vi "changeMonitorState.vi"(8 "error in (no error)":errorcluster, 10 "State":u16, 11 "Subnet in":refnum<class "Subnet.lvclass">) -> (0 "error out":errorcluster, 3 "Subnet out":refnum<class "Subnet.lvclass">)   [LabVIEW 2016, in "Subnet.lvclass"]
uses:
  Subnet.lvclass
  Subnet.lvclass/Subnet.ctl
  Common_RT_ILC/ILC/ILC.lvclass/ILC.ctl
  Common_RT_MTILC/MTILC/MTILC.lvclass
  D:/Code/Common_RT_ILC/ILC/ILC.lvclass
  Common_RT_MDILC/MDILC/MDILC.lvclass
  Common_RT_MIILC/MIILC/MIILC.lvclass
  Common_RT_Modbus/IModbus/IModbus.lvclass
  Common_RT_ILC/ILC/ILC.lvclass
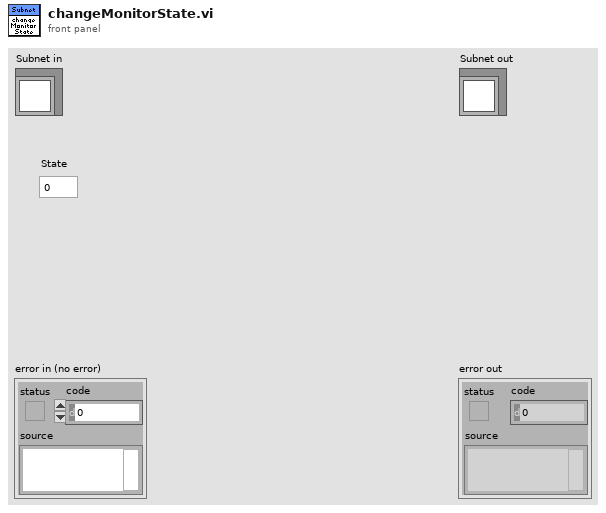
[diagram p1: front panel]
types:
  T1 = typedef "RTILC.lvlib/ILCData.ctl" = cluster{"Constants":T2, "Command":T3, "Telemetry":T5, "Responses":T6, "Timings":T8}
  T2 = typedef "RTILC.lvlib/ILCConstants.ctl" = cluster{"Subnet":u8, "Address":u8}
  T3 = typedef "RTILC.lvlib/ILCCommand.ctl" = cluster{"ILCMode":u16, "TemporaryAddress":u8, "ADCScanRate":T4, "ADCChannel":u8, "ADCOffset":sgl, "ADCSensitivity":sgl}
  T4 = typedef "RTILC.lvlib/ILCScanRates.ctl" = u8
  T5 = typedef "RTILC.lvlib/ILCTelemetry.ctl" = cluster{"UniqueID":u64, "FirmwareType":u8, "NetworkNodeType":u8, "ILCOption":u8, "NetworkNodeOption":u8, "MajorRevision":u8, "MinorRevision":u8, "FirmwareName":string, "ILCMode":u16, "MajorFault":bool, "MinorFault":bool, "FaultOverride":bool, "UniqueIDCRCMismatch":bool, "AppTypeNodeTypeMismatch":bool, "AppMissing":bool, "AppCRCMismatch":bool, "TEDSNotFound":bool, "TEDS1Mismatch":bool, "TEDS2Mismatch":bool, "WatchdogResetDetected":bool, "BrownoutDetected":bool, "EventTrapResetDetected":bool, "TemporaryAddress":u8, "ADCScanRate":T4, "DAC1":u16, "DAC2":u16, "DAC3":u16, "DAC4":u16, "MainADCCalibrationK":sgl[], "MainSensorOffset":sgl[], "MainSensorSensitivity":sgl[], "BackupADCCalibrationK":sgl[], "BackupSensorOffset":sgl[], "BackupSensorSensitivity":sgl[]}
  T6 = typedef "RTILC.lvlib/ILCResponses.ctl" = cluster{"ReportServerID":T7, "ReportServerStatus":T7, "ILCMode":T7, "SetTemporaryAddress":T7, "Reset":T7, "ADCScanRate":T7, "ADCOffsetSensitivity":T7, "ReadDAC":T7, "ReadCalibration":T7}
  T7 = typedef "RTModbus.lvlib/ExceptionCodes.ctl" = u16
  T8 = typedef "RTILC.lvlib/ILCTimings.ctl" = cluster{"ADCOffsetSensitivity":u32, "ADCScanRate":u32, "ILCMode":u32, "ReadCalibration":u32, "ReportServerID":u32, "ReportServerStatus":u32, "Reset":u32, "SetTemporaryAddress":u32}
  T9 = typedef "RTModbus.lvlib/TxFrame.ctl" = cluster{"Data":u8[], "WaitForTrigger":bool, "WaitForRx":u16, "TriggerIRQ":bool, "DelayMicroseconds":u16, "DelayMilliseconds":u16, "Timestamp":bool}
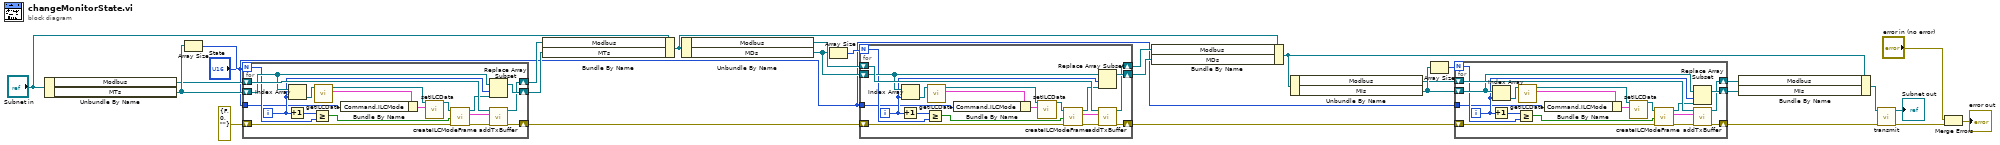
[diagram p0: block diagram]
diagram:
  n1 = Unbundle By Name("Subnet in") -> ("Modbus"=w19:refnum<class "IModbus.lvclass">, "MTs"=w20:refnum<class "MTILC.lvclass">[])
  n2 = Array Size(array=w20) -> (size(s)=w21:i32)
  n3 = for {
    N: w21 -> [w31]
    shift-right: [w37] -> w22
    shift-left: w19 -> [w42]
    shift-right: [w38] -> w23
    shift-left: w20 -> [w40]
    shift-right: [w35] -> w5
    shift-left: errorcluster {"status"=FALSE, "code"=0, "source"=""} ("error out") -> [w34]
    tunnel: "State" -> [w29]
    i -> [w33]
    n4 = Increment(x=w33) -> (x+1=w32:i32)
    n5 = Index Array(array=w40, index=w33) -> (element=w41:refnum<class "MTILC.lvclass">)
    n6 = Greater Or Equal?(x=w32, y=w31) -> (x >= y?=w30:bool)
    n7 = call "getILCData.vi"("ILC in"=w41) -> ("ILCData"=w46:T1, "ILC out"=w47:refnum<class "MTILC.lvclass">)  [unwired: 9 in]
    n8 = Bundle By Name(cluster=w46, "Command.ILCMode"=w29) -> (w45:T1)
    n9 = call "setILCData.vi"("ILCData"=w45, "ILC in"=w47) -> ("ILC out"=w44:refnum<class "MTILC.lvclass">)  [unwired: 9 in]
    n10 = call "createILCModeFrame.vi"("error in (no error)"=w34, "TriggerIRQ"=w30, "ILC in"=w44) -> ("error out"=w36:errorcluster, "TxFrame"=w43:T9, "ILC out"=w39:refnum<class "MTILC.lvclass">)  [unwired: 6 in]
    n11 = Replace Array Subset(array=w40, new element=w39, index=w33) -> (w38:refnum<class "MTILC.lvclass">[])
    n12 = call-dynamic "addTxBuffer.vi"("error in (no error)"=w36, "TxFrame"=w43, "IModbus in"=w42) -> ("error out"=w35:errorcluster, "IModbus out"=w37:refnum<class "IModbus.lvclass">)  [unwired: 7 in]
  }
  n13 = Bundle By Name(cluster="Subnet in", "Modbus"=w22, "MTs"=w23) -> (w13:refnum<class "Subnet.lvclass">)
  n14 = Unbundle By Name(w13) -> ("Modbus"=w18:refnum<class "IModbus.lvclass">, "MDs"=w17:refnum<class "MDILC.lvclass">[])
  n15 = Array Size(array=w17) -> (size(s)=w16:i32)
  n16 = for {
    N: w16 -> [w50]
    shift-right: [w56] -> w15
    shift-left: w18 -> [w61]
    shift-right: [w57] -> w14
    shift-left: w17 -> [w59]
    shift-right: [w54] -> w6
    shift-left: w5 -> [w53]
    tunnel: "State" -> [w48]
    i -> [w52]
    n17 = Increment(x=w52) -> (x+1=w51:i32)
    n18 = Index Array(array=w59, index=w52) -> (element=w60:refnum<class "MDILC.lvclass">)
    n19 = Greater Or Equal?(x=w51, y=w50) -> (x >= y?=w49:bool)
    n20 = call "getILCData.vi"("ILC in"=w60) -> ("ILCData"=w65:T1, "ILC out"=w66:refnum<class "MDILC.lvclass">)  [unwired: 9 in]
    n21 = Bundle By Name(cluster=w65, "Command.ILCMode"=w48) -> (w64:T1)
    n22 = call "setILCData.vi"("ILCData"=w64, "ILC in"=w66) -> ("ILC out"=w63:refnum<class "MDILC.lvclass">)  [unwired: 9 in]
    n23 = call "createILCModeFrame.vi"("error in (no error)"=w53, "TriggerIRQ"=w49, "ILC in"=w63) -> ("error out"=w55:errorcluster, "TxFrame"=w62:T9, "ILC out"=w58:refnum<class "MDILC.lvclass">)  [unwired: 6 in]
    n24 = Replace Array Subset(array=w59, new element=w58, index=w52) -> (w57:refnum<class "MDILC.lvclass">[])
    n25 = call-dynamic "addTxBuffer.vi"("error in (no error)"=w55, "TxFrame"=w62, "IModbus in"=w61) -> ("error out"=w54:errorcluster, "IModbus out"=w56:refnum<class "IModbus.lvclass">)  [unwired: 7 in]
  }
  n26 = Bundle By Name(cluster=w13, "Modbus"=w15, "MDs"=w14) -> (w7:refnum<class "Subnet.lvclass">)
  n27 = Unbundle By Name(w7) -> ("Modbus"=w8:refnum<class "IModbus.lvclass">, "MIs"=w9:refnum<class "MIILC.lvclass">[])
  n28 = Array Size(array=w9) -> (size(s)=w10:i32)
  n29 = for {
    N: w10 -> [w69]
    shift-right: [w75] -> w11
    shift-left: w8 -> [w80]
    shift-right: [w76] -> w12
    shift-left: w9 -> [w78]
    shift-right: [w73] -> w4
    shift-left: w6 -> [w72]
    tunnel: "State" -> [w67]
    i -> [w71]
    n30 = Increment(x=w71) -> (x+1=w70:i32)
    n31 = Index Array(array=w78, index=w71) -> (element=w79:refnum<class "MIILC.lvclass">)
    n32 = Greater Or Equal?(x=w70, y=w69) -> (x >= y?=w68:bool)
    n33 = call "getILCData.vi"("ILC in"=w79) -> ("ILCData"=w84:T1, "ILC out"=w85:refnum<class "MIILC.lvclass">)  [unwired: 9 in]
    n34 = Bundle By Name(cluster=w84, "Command.ILCMode"=w67) -> (w83:T1)
    n35 = call "setILCData.vi"("ILCData"=w83, "ILC in"=w85) -> ("ILC out"=w82:refnum<class "MIILC.lvclass">)  [unwired: 9 in]
    n36 = call "createILCModeFrame.vi"("error in (no error)"=w72, "TriggerIRQ"=w68, "ILC in"=w82) -> ("error out"=w74:errorcluster, "TxFrame"=w81:T9, "ILC out"=w77:refnum<class "MIILC.lvclass">)  [unwired: 6 in]
    n37 = Replace Array Subset(array=w78, new element=w77, index=w71) -> (w76:refnum<class "MIILC.lvclass">[])
    n38 = call-dynamic "addTxBuffer.vi"("error in (no error)"=w74, "TxFrame"=w81, "IModbus in"=w80) -> ("error out"=w73:errorcluster, "IModbus out"=w75:refnum<class "IModbus.lvclass">)  [unwired: 7 in]
  }
  n39 = Bundle By Name(cluster=w7, "Modbus"=w11, "MIs"=w12) -> (w3:refnum<class "Subnet.lvclass">)
  n40 = call "transmit.vi"("error in (no error)"=w4, "Subnet in"=w3) -> ("error out"=w25:errorcluster, "Subnet out"=→"Subnet out":refnum<class "Subnet.lvclass">)  [unwired: 8 in]
  n41 = Merge Errors("error in (no error)", w25) -> (→"error out":errorcluster)
